vi "host_with_subvis_timed_pulse.vi"() -> ()   [LabVIEW 2015]
uses:
  <vilib>/userdefined/High Color/nirio_resource_hc.ctl
  <vilib>/DAQmx/create/channels.llb/DAQmx Create Channel (CO-Pulse Generation-Time).vi
  <vilib>/DAQmx/configure/timing.llb/DAQmx Timing (Implicit).vi
  <vilib>/DAQmx/configure/trigger.llb/DAQmx Start Trigger (Digital Edge).vi
  <instrlib>/niSync/niSync.llb/niSync Initialize (IVI).vi
  <vilib>/FPGAPlugInAG/Dynamic/niLvFpga_Close_Dynamic.vi
  <vilib>/rvi/interface/nirviCloseFPGA/nirviCloseFPGA.xnode
  <vilib>/Utility/file.llb/Write Delimited Spreadsheet (DBL).vi
panel:
  in  "Analog High Pass Filter":bool
  in  "High Pass Filter K":u16=11 format="%b"
  out "Waveform Graph 2":waveform(i16)(graph)
  in  "AI to plot":i32
  in  "trigger  delay":u64
  in  "destination terminal":string(combo)="PXI_Trig0"
  out "Waveform Graph":waveform(dbl)(graph)
  out "Interleaved Raw Data":u64[](array[numeric])
  out "Counts":i16[][](array[numeric])
  out "Voltage":dbl[][](array[numeric])
  in  "num samples":u64=1000
  in  "FPGA name":T1 caption="RIO Device"
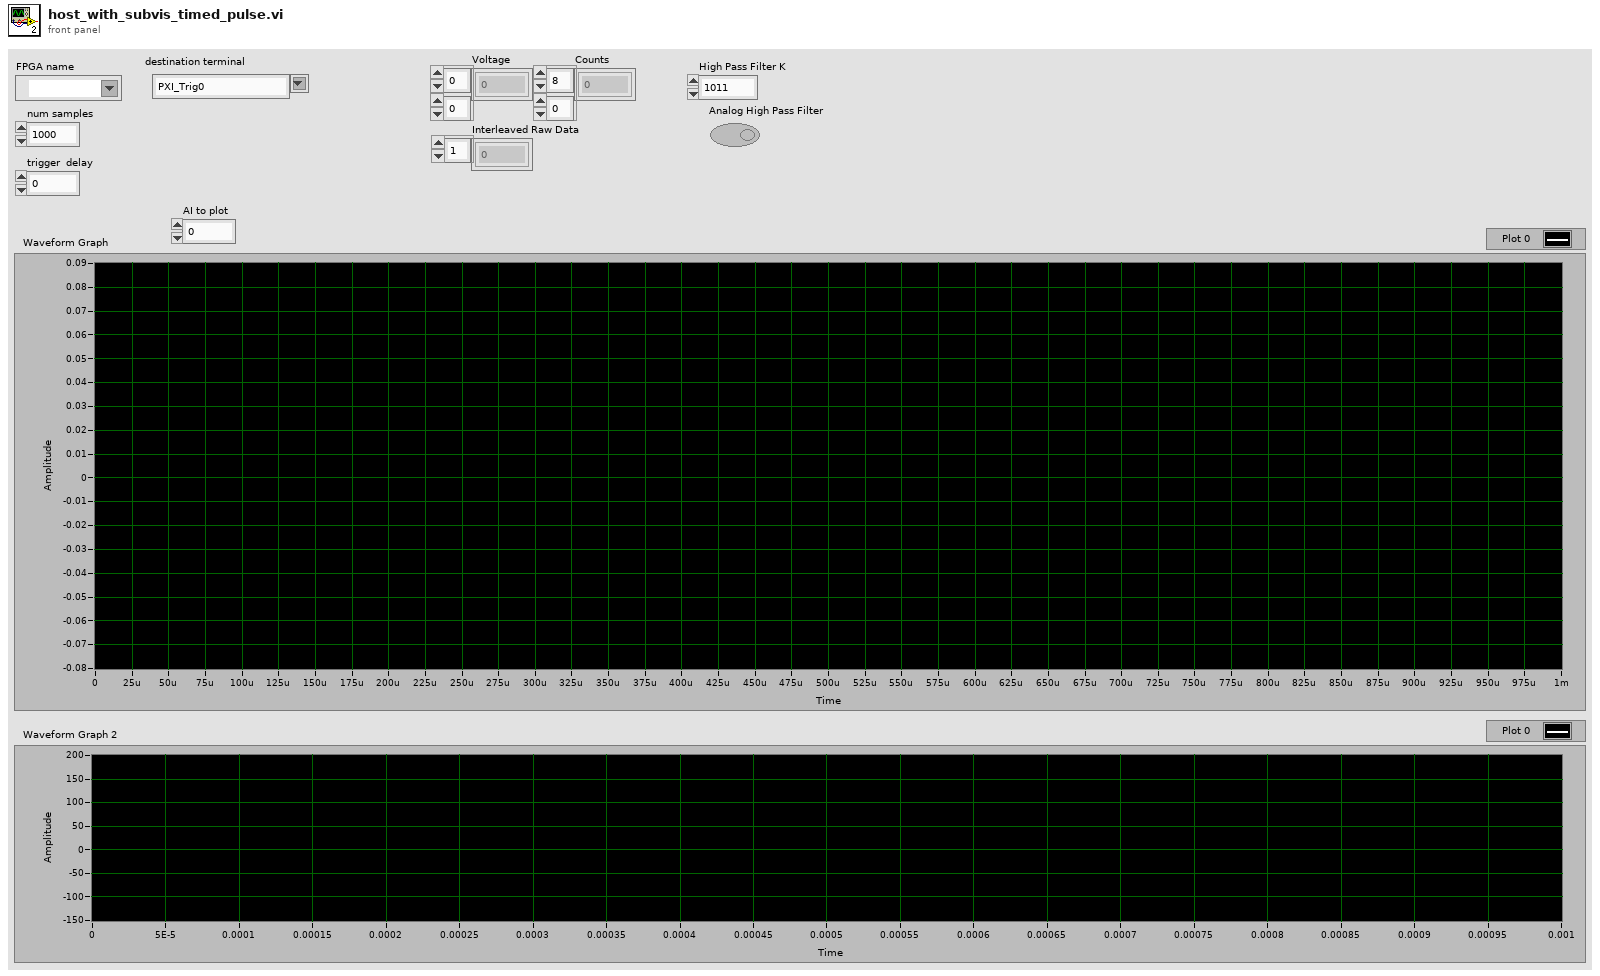
[diagram p1: front panel]
types:
  T1 = typedef "nirio_resource_hc.ctl" = tag
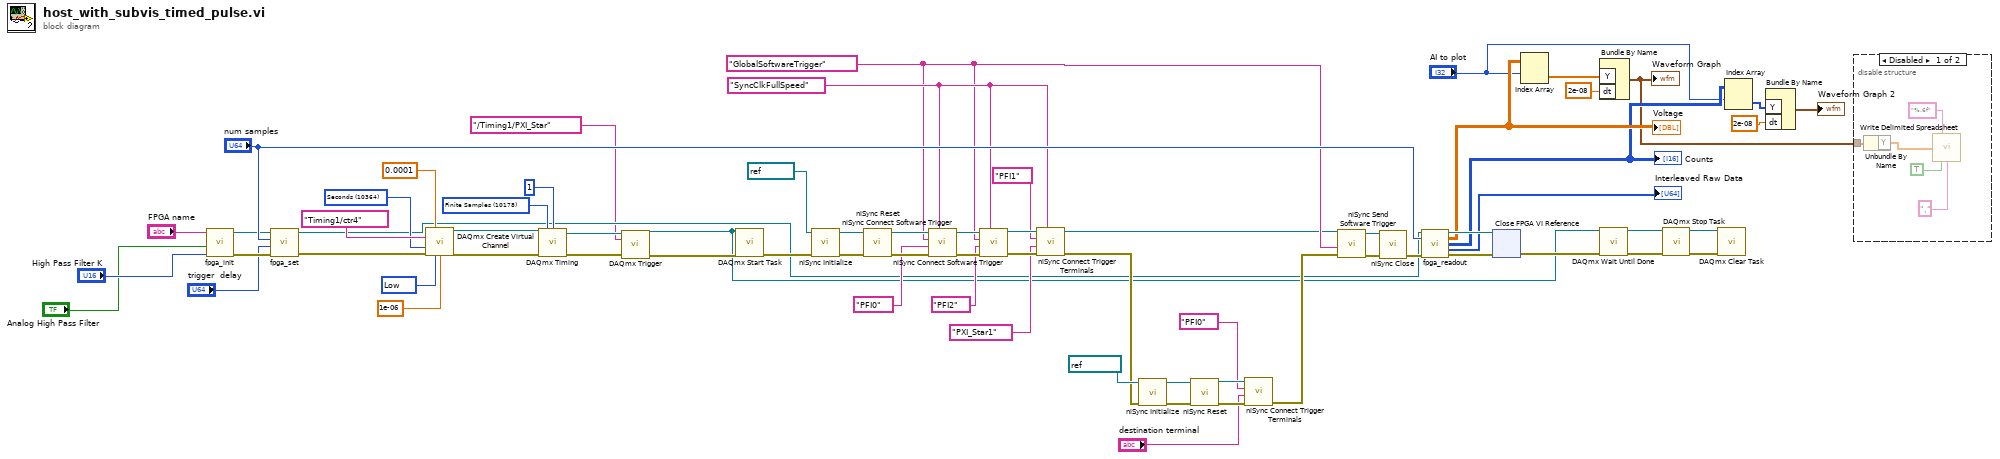
[diagram p0: block diagram]
diagram:
  w15 = 10178 items=["Finite Samples"=10178, "Continuous Samples"=10123, "Hardware Timed Single Point"=12522] ("sample mode")
  w17 = 10214 items=["High"=10192, "Low"=10214] ("idle state")
  w19 = 10364 items=["Seconds"=10364] ("units")
  w33 = "SyncClkFullSpeed" ("synchronization clock")
  w32 = "GlobalSoftwareTrigger" ("source terminal")
  n1 = call "fpga_init.vi"("High Pass Filter K"="High Pass Filter K", "Analog High Pass Filter"="Analog High Pass Filter", "FPGA name"="FPGA name") -> ("error out"=w69:errorcluster, "FPGA VI Reference Out"=w57:refnum<k20>)  [unwired: 7 in]
  n2 = call "fpga_set.vi"("error in"=w69, "trigger  delay"="trigger  delay", "num samples"="num samples", "FPGA VI Reference In"=w57) -> ("error out"=w10:errorcluster, "FPGA VI Reference Out"=w8:refnum<k20>)  [unwired: 6 in]
  n3 = call-poly <vilib>:"DAQmx Create Virtual Channel.vi"("high time"=0.0001, "counter"=tag "Timing1/ctr4", "units"=w19, "error in"=w10, "idle state"=w17, "initial delay"=1e-06) -> ("task out"=w21:refnum<k21>, "error out"=w22:errorcluster)  [unwired: 8 in]
  n4 = call-poly <vilib>:"DAQmx Timing.vi"("task/channels in"=w21, "sample mode"=w15, "samples per channel"=1, "error in"=w22) -> ("task out"=w13:refnum<k21>, "error out"=w12:errorcluster)  [unwired: 10 in]
  n5 = call-poly <vilib>:"DAQmx Trigger.vi"("task/channels in"=w13, "source"=tag "/Timing1/PXI_Star", "error in"=w12) -> ("task out"=w5:refnum<k21>, "error out"=w11:errorcluster)  [unwired: 11 in]
  n6 = call <vilib>:"DAQmx Start Task.vi"("task/channels in"=w5, "error in"=w11) -> ("error out"=w9:errorcluster)  [unwired: 12 in, 1 out]
  n7 = call-poly <instrlib>:"niSync Initialize.vi"("error in (no error)"=w9, "resource name"=refnum<k15> "Sync") -> ("error out"=w49:errorcluster, "instrument handle out"=w50:refnum<k15>)  [unwired: 8 in]
  n8 = call <instrlib>:"niSync Reset.vi"("error in (no error)"=w49, "instrument handle"=w50) -> ("error out"=w41:errorcluster, "instrument handle out"=w40:refnum<k15>)  [unwired: 8 in]
  n9 = call <instrlib>:"niSync Connect Software Trigger.vi"("synchronization clock"=w33, "error in (no error)"=w41, "destination terminal"="PFI0", "source terminal"=w32, "instrument handle"=w40) -> ("error out"=w38:errorcluster, "instrument handle out"=w39:refnum<k15>)  [unwired: 5 in]
  n10 = call <instrlib>:"niSync Connect Software Trigger.vi"("synchronization clock"=w33, "error in (no error)"=w38, "destination terminal"="PFI2", "source terminal"=w32, "instrument handle"=w39) -> ("error out"=w36:errorcluster, "instrument handle out"=w37:refnum<k15>)  [unwired: 5 in]
  n11 = call <instrlib>:"niSync Connect Trigger Terminals.vi"("synchronization clock"=w33, "error in (no error)"=w36, "destination terminal"="PXI_Star1", "source terminal"="PFI1", "instrument handle"=w37) -> ("error out"=w27:errorcluster, "instrument handle out"=w25:refnum<k15>)  [unwired: 5 in]
  n12 = call-poly <instrlib>:"niSync Initialize.vi"("error in (no error)"=w27, "resource name"=refnum<k15> "Sync1") -> ("error out"=w47:errorcluster, "instrument handle out"=w48:refnum<k15>)  [unwired: 8 in]
  n13 = call <instrlib>:"niSync Reset.vi"("error in (no error)"=w47, "instrument handle"=w48) -> ("error out"=w34:errorcluster, "instrument handle out"=w35:refnum<k15>)  [unwired: 8 in]
  n14 = call <instrlib>:"niSync Connect Trigger Terminals.vi"("error in (no error)"=w34, "destination terminal"="destination terminal", "source terminal"="PFI0", "instrument handle"=w35) -> ("error out"=w26:errorcluster)  [unwired: 6 in, 1 out]
  n15 = call <instrlib>:"niSync Send Software Trigger.vi"("error in (no error)"=w26, "source terminal"=w32, "instrument handle"=w25) -> ("error out"=w51:errorcluster, "instrument handle out"=w52:refnum<k15>)  [unwired: 7 in]
  n16 = call <instrlib>:"niSync Close.vi"("error in (no error)"=w51, "instrument handle"=w52) -> ("error out"=w66:errorcluster)  [unwired: 9 in]
  n17 = call "fpga_readout.vi"("FPGA VI Reference In"=w8, "samples"="num samples", "error in"=w66) -> ("FPGA VI Reference Out"=w60:refnum<k20>, "Voltage"=w58:dbl[][], "Counts"=w55:i16[][], "Interleaved Raw Data"=→"Interleaved Raw Data":u64[], "error out"=w63:errorcluster)  [unwired: 8 in]
  "Voltage" <- w58
  "Counts" <- w55
  n18 = xnode "Close FPGA VI Reference"("FPGA VI Reference In"=w60, "error in"=w63) -> ("error out"=w6:errorcluster)
  n19 = Index Array(array=w58, index (row)="AI to plot") -> (element=w61:dbl[])  [unwired: 1 in]
  n20 = Bundle By Name("Y"=w61, "dt"=2e-08) -> (w2:waveform(dbl))  [unwired: 1 in]
  "Waveform Graph" <- w2
  n21 = call <vilib>:"DAQmx Wait Until Done.vi"("task/channels in"=w5, "error in"=w6) -> ("task out"=w45:refnum<k21>, "error out"=w44:errorcluster)  [unwired: 12 in]
  n22 = call <vilib>:"DAQmx Stop Task.vi"("task/channels in"=w45, "error in"=w44) -> ("task out"=w43:refnum<k21>, "error out"=w42:errorcluster)  [unwired: 12 in]
  n23 = call <vilib>:"DAQmx Clear Task.vi"("task in"=w43, "error in"=w42) -> ()  [unwired: 13 in, 1 out]
  n24 = Index Array(array=w55, index (row)="AI to plot") -> (element=w54:i16[])  [unwired: 1 in]
  n25 = Bundle By Name("Y"=w54, "dt"=2e-08) -> (→"Waveform Graph 2":waveform(i16))  [unwired: 1 in]
  n26 = disable-structure shown="Disabled" {
    disable-tunnel: w2 -> [w73 _]
    frame Disabled {
      n27 = Unbundle By Name(w73) -> ("Y"=w74:dbl[])
      n28 = call-poly <vilib>:"Write Delimited Spreadsheet.vi"("format (%.3f)"="%.6f", "1D data"=w74, "transpose? (F)"=TRUE, "delimiter (\\t)"="," ("delimiter (\\t)")) -> ()  [unwired: 10 in, 2 out]
    }
    frame Enabled {
    }
  }
